vi "Error Converter (ErrCode or Status).vi"(8 "error in (no error)":errorcluster, 11 "StatusInfo":T1) -> (0 "error out":errorcluster)   [LabVIEW 2016, in "fgt_SDK.lvlib"]
doc: "Internal use only"
uses:
  fgt_SDK.lvlib
  TypeDefs/fgt_ERROR_CODE.ctl
  TypeDefs/fgt_INSTRUMENT_TYPE.ctl
  TypeDefs/fgt_STATUS_INFO.ctl
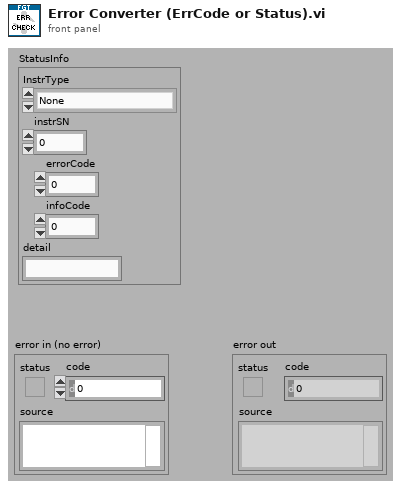
[diagram p1: front panel]
types:
  T1 = typedef "fgt_SDK.lvlib/fgt_STATUS_INFO.ctl" = cluster{"InstrType":T2, "instrSN":u16, "errorCode":u8, "infoCode":u8, "detail":string}
  T2 = typedef "fgt_SDK.lvlib/fgt_INSTRUMENT_TYPE.ctl" = enum32{"None", "MFCS", "MFCS_EZ", "FRP", "LineUP", "IPS"}
  T3 = typedef "fgt_SDK.lvlib/fgt_ERROR_CODE.ctl" = enum8{"OK", "USB_error", "Wrong_command", "No_Module_at_index", "Wrong_module", "Module_is_sleep", "Master_error", "Failed_init_all_instr", "Wrong_parameter", "Overpressure", "Underpressure", "No_instr_found", "No_modules_found", "No_pressure_controller_found", "Dll_dependency_error"}
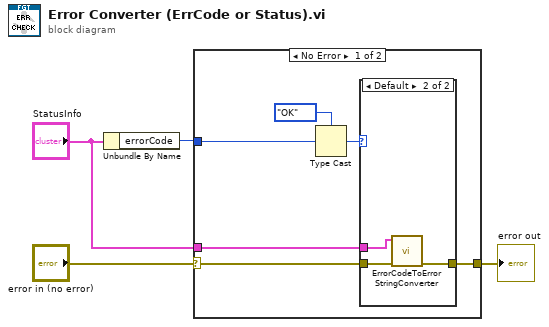
[diagram p0: block diagram]
diagram:
  n1 = Unbundle By Name("StatusInfo") -> ("errorCode"=w2:u8)
  n2 = case shown="No Error" "error in (no error)" {
    selector: "error in (no error)" -> [w10 w15]
    tunnel: [w9 w15] -> w3
    tunnel: w2 -> [w7 _]
    tunnel: "StatusInfo" -> [w5 _]
    frame No Error {
      n3 = Type Cast(type=fgt_ERROR_CODE."OK" ("fgt_ERROR_CODE"), x=w7) -> (*(type *) &x=w6:T3)
      n4 = case shown="Default" w6 {
        tunnel: w10 -> [w11 w14]
        tunnel: [w11 w13] -> w9
        tunnel: w5 -> [_ w12]
        frame "OK" {
        }
        frame Default {
          n5 = call "ErrorCodeToErrorStringConverter.vi"("error in (no error)"=w14, "StatusInfo"=w12) -> ("error out"=w13:errorcluster)  [unwired: 9 in]
        }
      }
    }
    frame Error {
    }
  }
  "error out" <- w3
